vi "SetFlags.vi"(8 "error in (no error)":errorcluster, 10 "Flags":T1, 11 "Window in":refnum<class "Window.lvclass">) -> (0 "error out":errorcluster, 3 "Window out":refnum<class "Window.lvclass">)   [LabVIEW 2020, in "GLF.lvlib" / "Window.lvclass"]
uses:
  Window.lvclass
  Window.lvclass/Window.ctl
  Flags--cluster.ctl
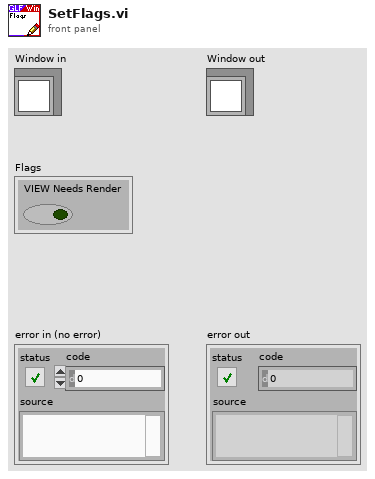
[diagram p1: front panel]
types:
  T1 = typedef "GLF.lvlib/Window.lvclass/Flags--cluster.ctl" = cluster{"VIEW Needs Render":bool}
  T2 = typedef "GLF.lvlib/Window.lvclass/DVR--cluster.ctl" = cluster{"SDL_Window *":T3, "Window ID":T4, "SDL_Renderer *":T5, "Event Interface":refnum<class "WindowEventInterface.lvclass">, "VIEW":refnum<class "IAmVIEW.lvclass">, "Flags":T1}
  T3 = typedef "SDL3.lvlib/Video.lvlib/SDL_Window--pointer.ctl" = i64
  T4 = typedef "SDL3.lvlib/Video.lvlib/WindowID--integer.ctl" = u32
  T5 = typedef "SDL3.lvlib/Render.lvlib/SDL_Renderer--pointer.ctl" = i64
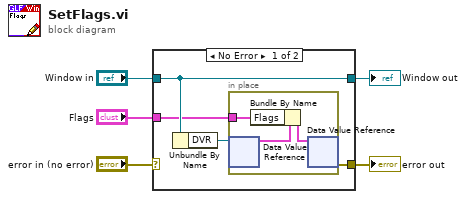
[diagram p0: block diagram]
diagram:
  n1 = case shown="No Error" "error in (no error)" {
    selector: "error in (no error)" -> [_ w13]
    tunnel: "Window in" -> [w9 w14]
    tunnel: [w7 w13] -> w3
    tunnel: [w9 w14] -> w2
    tunnel: "Flags" -> [w6 _]
    frame No Error {
      n2 = Unbundle By Name(w9) -> ("DVR"=w8:refnum<data-value>)
      n3 = in-place {
        in-place-border: w6 -> [w10]
        n4 = in-place-dvr #1(w8) -> (w12:T2)  [unwired: 1 out]
        n5 = Bundle By Name(cluster=w12, "Flags"=w10) -> (w11:T2)
        n6 = in-place-dvr #1(w11) -> (w7:errorcluster)  [unwired: 1 out]
      }
    }
    frame Error {
    }
  }
  "Window out" <- w2
  "error out" <- w3
